vi "test.vi"() -> ()   [LabVIEW 2010, in "AnalysisRAPS.lvclass"]
uses:
  AnalysisRAPS.lvclass
panel:
  out "x+y":i32[](array[numeric])
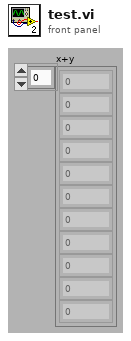
[diagram p1: front panel]
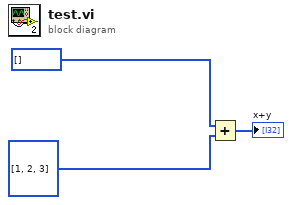
[diagram p0: block diagram]
diagram:
  n1 = Add(x=i32[] [], y=i32[] [1, 2, 3]) -> (x+y=→"x+y":i32[])
